vi "SimpleSerialWriteAndRead.vi"() -> ()   [LabVIEW 2020]
doc: "LabVIEW example of write/read serial communication . Transmitted data in the form of single-byte messages. Works with Arduino Uno with SimpeSerialWriteAndRead_Arduino code. Comments in Polish."
uses:
  58620be1-59da-469e-9dfd-42fdba33ff9f.vi
  <vilib>/Instr/_visa.llb/VISA Configure Serial Port (Instr).vi
panel:
  out "#bytesPort":u32 caption="Liczba bajtów w buforze \nna porcie szeregowym"
  out "readBuffer":string caption="Odczytane dane"
  in  "writeBuffer":string(combo)="a" caption="Dane do wysłania"
  out "#returnByte":u32 caption="Liczba zapisanych bajtów"
  in  "stop bits (10: 1 bit)":u16(ring)=10 caption="Liczba bitów stopu" items=["1.0"=10, "1.5"=15, "2.0"=20]
  in  "timeout (10sec)":u32=10000 caption="Timeout"
  in  "parity (0:none)":enum16{"None", "Odd", "Even", "Mark", "Space"}(ring) caption="Bit parzystości"
  in  "data bits (8)":u16=8 caption="Liczba bitów w ramce"
  in  "baud rate (9600)":u32=9600 caption="Szybkość transmisji"
  in  "VISA resource name":refnum<visa-resource-name>="COM7" caption="Port do komunikacji"
  in  "stop":bool
  # "Odczyt danych"
  # "Zapis danych"
  # "Konfiguracja"
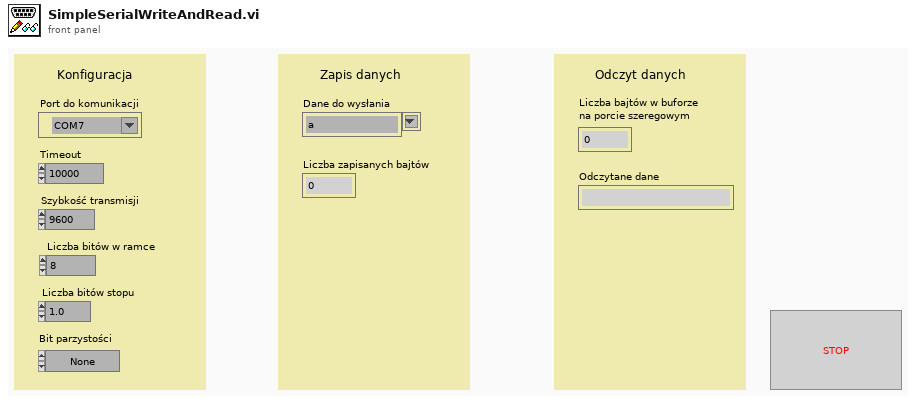
[diagram p1: front panel]
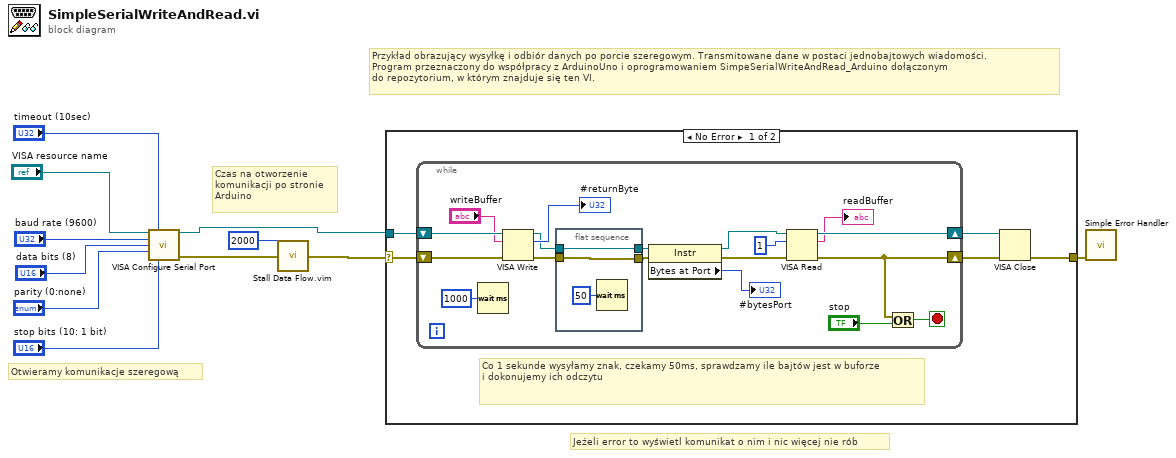
[diagram p0: block diagram]
diagram:
  # "Przykład obrazujący wysyłkę i odbiór danych po porcie szeregowym. Transmitowane dane w postaci jednobajtowych wiadomości. \nProgram przeznaczony do współpracy z ArduinoUno i oprogramowaniem SimpeSerialWriteAndRead_Arduino dołączonym \ndo repozytorium, w którym znajduje się ten VI."
  # "Jeżeli error to wyświetl komunikat o nim i nic więcej nie rób"
  # "Czas na otworzenie \nkomunikacji po stronie\nArduino"
  # "Otwieramy komunikacje szeregową"
  n1 = call-poly "VISA Configure Serial Port"("VISA resource name"="VISA resource name", "timeout (10sec)"="timeout (10sec)", "baud rate (9600)"="baud rate (9600)", "data bits (8)"="data bits (8)", "parity (0:none)"="parity (0:none)", "stop bits (10: 1 bit)"="stop bits (10: 1 bit)") -> ("VISA resource name out"=w1:refnum<visa-resource-name>, "error out"=w4:errorcluster)  [unwired: 8 in]
  n2 = call "Stall Data Flow.vim"("value in"=w4, "milliseconds to wait"=u32 2000) -> ("value out"=w3:errorcluster)  [unwired: 1 out]
  n3 = case shown="No Error" w3 {
    selector: w3 -> [w15 w38]
    tunnel: w1 -> [w16 _]
    tunnel: [w12 w38] -> w5
    frame No Error {
      # "Co 1 sekunde wysyłamy znak, czekamy 50ms, sprawdzamy ile bajtów jest w buforze \ni dokonujemy ich odczytu"
      n4 = while {
        shift-right: [w27] -> w13
        shift-left: w15 -> [w33]
        shift-right: [w25] -> w14
        shift-left: w16 -> [w32]
        stop <- w29 stop-if-true
        n5 = Wait (ms)(milliseconds to wait=u32 1000) -> ()  [unwired: 1 out]
        n6 = VISA Write(VISA resource name=w32, write buffer="writeBuffer", error in (no error)=w33) -> (VISA resource name out=w22:refnum<visa-resource-name>, return count=→"#returnByte":u32, error out=w20:errorcluster)
        n7 = flat-sequence {
          tunnel: w22 -> [w37]
          tunnel: [w37] -> w21
          tunnel: w20 -> [w36]
          tunnel: [w36] -> w19
          frame #0 {
            n8 = Wait (ms)(milliseconds to wait=u32 50) -> ()  [unwired: 1 out]
          }
        }
        n9 = property class="Instr"(reference=w21, error in=w19) -> (reference out=w26:refnum<visa-resource-name>, error out=w28:errorcluster, "Bytes at Port"=→"#bytesPort":u32)
        n10 = VISA Read(VISA resource name=w26, byte count=u32 1, error in (no error)=w28) -> (VISA resource name out=w25:refnum<visa-resource-name>, read buffer=→"readBuffer":string, error out=w27:errorcluster)  [unwired: 1 out]
        n11 = Or(x=w27, y="stop") -> (x .or. y?=w29:bool)
      }
      n12 = VISA Close(VISA resource name=w14, error in (no error)=w13) -> (error out=w12:errorcluster)
    }
    frame Error {
    }
  }
  n13 = call <vilib>:"Simple Error Handler.vi"("error in (no error)"=w5) -> ()  [unwired: 4 in, 5 out]
